vi "SetPower.vi"(8 "error in (no error)":errorcluster, 9 "Numeric":dbl, 10 "PowerType":enum16{"Itech", "Keysight"}(ring), 11 "Execute":refnum<class "Execute.lvclass">) -> (0 "error out":errorcluster, 3 "Execute":refnum<class "Execute.lvclass">)   [LabVIEW 2018, in "QMH_Class.lvlib" / "TestManager.lvlib" / "Execute.lvclass"]
uses:
  Execute.lvclass
  Execute.lvclass/Execute.ctl
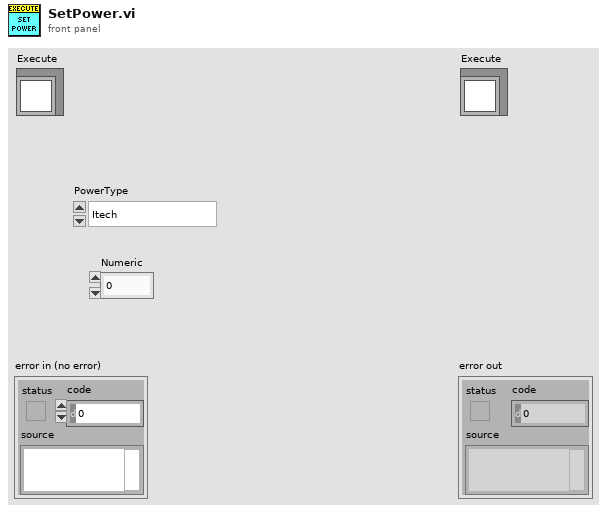
[diagram p1: front panel]
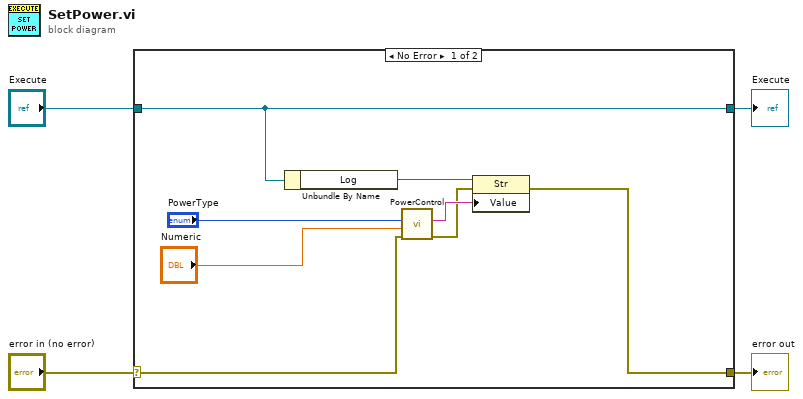
[diagram p0: block diagram]
diagram:
  n1 = case shown="No Error" "error in (no error)" {
    selector: "error in (no error)" -> [w7 w14]
    tunnel: [w5 w14] -> w3
    tunnel: [w10 w13] -> w1
    tunnel: "Execute" -> [w10 w13]
    frame No Error {
      n2 = Unbundle By Name(w10) -> ("Log"=w12:refnum<vi>)
      n3 = call "PowerControl.vi"("error in (no error)"=w7, "Numeric"="Numeric", "PowerType"="PowerType") -> ("error out"=w6:errorcluster, "Fb"=w11:string)  [unwired: 7 in]
      n4 = property class="Str"(reference=w12, error in=w6, "Value"=w11) -> (error out=w5:errorcluster)  [unwired: 1 out]
    }
    frame Error {
    }
  }
  "error out" <- w3
  "Execute" <- w1
